vi "Read Adu Device.vi"(6 "#BytesToRead":u32, 7 "Timeout":u32, 8 "error in (no error)":errorcluster, 11 "Device Handle":u32) -> (0 "error out":errorcluster, 1 "Read Buffer":string, 2 "function return":i32, 3 "Device Handle out":u32, 4 "#BytesRead":u32)   [LabVIEW 2015, in "AduHid.lvlib"]
doc: "int __stdcall ReadAduDevice(void * hDevice, \n void * lpBuffer, \n unsigned long nNumberOfBytesToRead,\n unsigned long * lpNumberOfBytesRead,\n unsigned long iTimeout);"
uses:
  AduHid.lvlib
  Windows/SysWOW64/kernel32.dll
  AduHid.dll
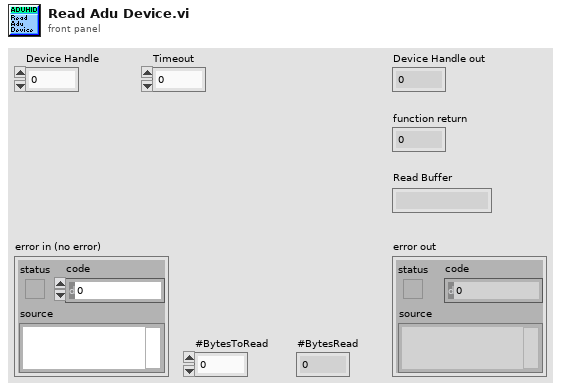
[diagram p1: front panel]
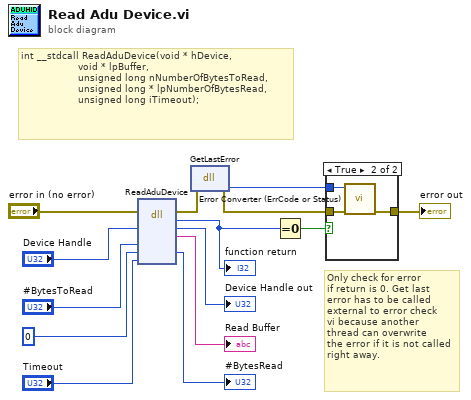
[diagram p0: block diagram]
diagram:
  # "Only check for error\nif return is 0. Get last\nerror has to be called\nexternal to error check\nvi because another\nthread can overwrite\nthe error if it is not called\nright away."
  # "int __stdcall ReadAduDevice(void * hDevice, \n                   void * lpBuffer, \n                   unsigned long nNumberOfBytesToRead,\n                   unsigned long * lpNumberOfBytesRead,\n                   unsigned long iTimeout);"
  n1 = dll-call lib="C:/Projects/CBTF Modules/Libraries/Ontrak ADU/API/AduHid.*" fn="ReadAduDevice"(error in="error in (no error)", "Device Handle"="Device Handle", "#BytesToRead"="#BytesToRead", "#BytesRead"=u32 0, "Timeout"="Timeout") -> (error out=w5:errorcluster, "return type"=w1:i32, "Device Handle"=→"Device Handle out":u32, "Read Buffer"=→"Read Buffer":string, "#BytesRead"=→"#BytesRead":u32)  [unwired: 5 in, 1 out]
  "function return" <- w1
  n2 = dll-call lib="C:/Windows/SysWOW64/kernel32.dll" fn="GetLastError"(error in=w5) -> (error out=w4:errorcluster, "return type"=w3:u32)  [unwired: 2 in, 1 out]
  n3 = Equal To 0?(x=w1) -> (x = 0?=w2:bool)
  n4 = case shown="True" w2 {
    tunnel: [w15 w18] -> w7
    tunnel: w4 -> [w15 w17]
    tunnel: w3 -> [_ w16]
    frame False {
    }
    frame True {
      n5 = call "Error Converter (ErrCode or Status).vi"("error in (no error)"=w17, "error code"=w16) -> ("error out"=w18:errorcluster)  [unwired: 9 in]
    }
  }
  "error out" <- w7
